vi "Load Resource File.vi"(8 "error in (no error)":errorcluster, 11 "Resource File":path) -> (0 "error out":errorcluster, 2 "File Type":string, 3 "Resources":T1[](array[typedef]))   [LabVIEW 2026, in "VILab.lvlib"]
uses:
  VILab.lvlib
  CTLs/Resource.ctl
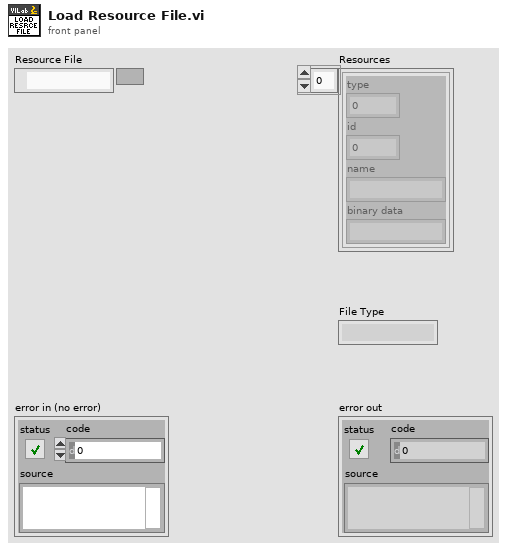
[diagram p1: front panel]
types:
  T1 = typedef "VILab.lvlib/Resource.ctl" = cluster{"type":u32, "id":i32, "name":string, "binary data":string}
  T2 = cluster{"type":u32, "id":i32, "name":string, "binary data":string}[]
  T3 = cluster{"type":u32, "id":i32, "name":string, "binary data":string}
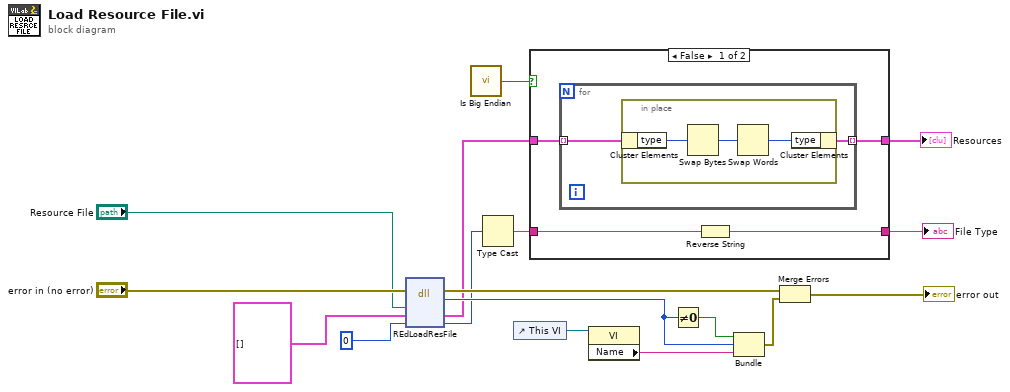
[diagram p0: block diagram]
diagram:
  n1 = dll-call lib="LabVIEW" fn="REdLoadResFile"(error in="error in (no error)", "resource binary file"="Resource File", "resources"=T2 [], 0) -> (error out=w17:errorcluster, w8:i32, "resources"=w4:T2, w5:i32)  [unwired: 3 in, 1 out]
  n2 = call "Is Big Endian.vi"() -> ("big endian"=w2:bool)
  n3 = Type Cast(x=w5) -> (*(type *) &x=w3:string)  [unwired: 1 in]
  n4 = control-ref of="This VI"() -> (w9:refnum<vi>)
  n5 = case shown="False" w2 {
    tunnel: w4 -> [w21 w28]
    tunnel: [w20 w28] -> w14
    tunnel: [w18 w27] -> w13
    tunnel: w3 -> [w19 w27]
    frame False {
      n6 = for {
        tunnel: w21 -> [w23] mode=indexing
        tunnel: [w22] -> w20 mode=indexing
        n7 = in-place {
          n8 = in-place-cluster #1(w23) -> ("type"=w26:u32)
          n9 = Swap Bytes(anything=w26) -> (byte swapped=w25:u32)
          n10 = Swap Words(1:w25) -> (0:w24:u32)
          n11 = in-place-cluster #1("type"=w24) -> (w22:T3)
        }
      }
      n12 = Reverse String(1:w19) -> (0:w18:string)
    }
    frame True {
    }
  }
  "Resources" <- w14
  "File Type" <- w13
  n13 = property class="VI"(reference=w9) -> ("Name"=w6:string)  [unwired: 1 in, 2 out]
  n14 = Not Equal To 0?(x=w8) -> (x != 0?=w7:bool)
  n15 = Bundle(w7, w8, "Name"=w6) -> (w16:cluster{bool, i32, "Name":string})  [unwired: 1 in]
  n16 = Merge Errors(w17, w16) -> (→"error out":errorcluster)
